vi "Startup - Read INI.vi"(8 "error IO":errorcluster, 11 "ini path":path) -> (0 "error out":errorcluster, 2 "Key Values":string[](array[string]), 3 "Key Names":string[](array[string]))   [LabVIEW 2010]
uses:
  <vilib>/Utility/config.llb/Read Key (String).vi
  <vilib>/Utility/config.llb/NI_LVConfig.lvlib
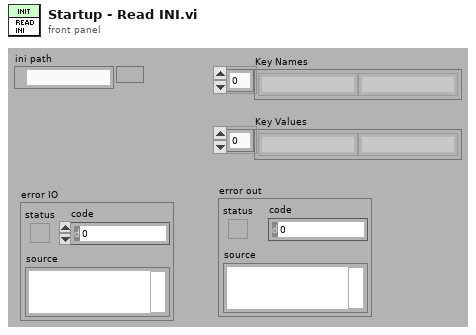
[diagram p1: front panel]
types:
  T1 = typedef "NI_LVConfig.lvlib/Config Data RefNum.ctl" = refnum<k1>
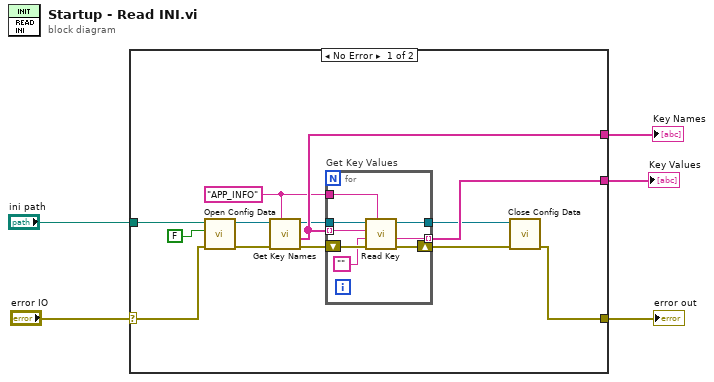
[diagram p0: block diagram]
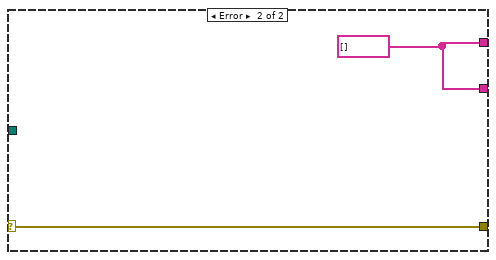
[diagram p2: hidden frame]
diagram:
  n1 = case shown="No Error" "error IO" {
    selector: "error IO" -> [w9 w28]
    tunnel: [w18 w27] -> w5
    tunnel: "ini path" -> [w17 _]
    tunnel: [w6 w28] -> w3
    tunnel: [w16 w27] -> w2
    frame No Error {
      w15 = "APP_INFO"
      n2 = call <vilib>:"Open Config Data.vi"("error in (no error)"=w9, "create file if necessary (T)"=FALSE ("create file if necessary? (T)"), "configuration file path"=w17) -> ("error out"=w12:errorcluster, "refnum"=w11:T1)  [unwired: 6 in, 1 out]
      n3 = call <vilib>:"Get Key Names.vi"("section"=w15, "error in (no error)"=w12, "refnum"=w11) -> ("error out"=w14:errorcluster, "key names"=w16:string[], "refnum out"=w13:T1)  [unwired: 5 in, 1 out]
      n4 = for "Get Key Values" {
        tunnel: w13 -> [w26]
        tunnel: w15 -> [w24]
        tunnel: w16 -> [w23] mode=indexing
        tunnel: [w21] -> w18 mode=indexing
        shift-right: [w20] -> w8
        shift-left: w14 -> [w25]
        tunnel: [w19] -> w7
        n5 = call-poly <vilib>:"Read Key.vi"("section"=w24, "error in (no error)"=w25, "default value"="", "key"=w23, "refnum"=w26) -> ("error out"=w20:errorcluster, "value"=w21:string, "refnum out"=w19:T1)  [unwired: 3 in, 1 out]
      }
      n6 = call <vilib>:"Close Config Data.vi"("error in (no error)"=w8, "refnum"=w7) -> ("error out"=w6:errorcluster)  [unwired: 8 in, 1 out]
    }
    frame Error {
      w27 = string[] [] ("key names")
    }
  }
  "Key Values" <- w5
  "error out" <- w3
  "Key Names" <- w2
